vi "Find overlattice using co-incident search.vi"(6 "Minimal Angle from GB plane":dbl, 7 "Minimal thickness of the grain (A)":dbl=0.05, 8 "Co-incidence Tolerance":dbl=0.05, 9 "Number of integers to search":i32=50, 10 "Mutual Viewing Angle":dbl[](array[numeric])=[0.0, 1.0, 0.0], 11 "Grain Boundary Macro Definition":T1={"Grain 1 Orientation"=[1.0, 0.0, 0.0], "Grain 2 Orientation"=[0.707, 0.707, 0.0], "Twist Angle (Deg)"=0.0}) -> (1 "Perpendicular to GB Plane, Lattice c":dbl[](array[numeric]), 2 "GB Plane 2, Lattice b":dbl[](array[numeric]), 3 "GB Plane 1, Lattice a":dbl[](array[numeric]))   [LabVIEW 2010]
panel:
  out "Angle (Degrees)":dbl
  out "deleted portion":dbl[](array[numeric])
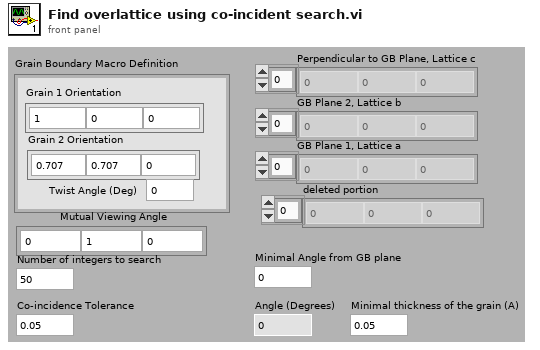
[diagram p1: front panel]
types:
  T1 = cluster{"Grain 1 Orientation":dbl[], "Grain 2 Orientation":dbl[], "Twist Angle (Deg)":dbl}
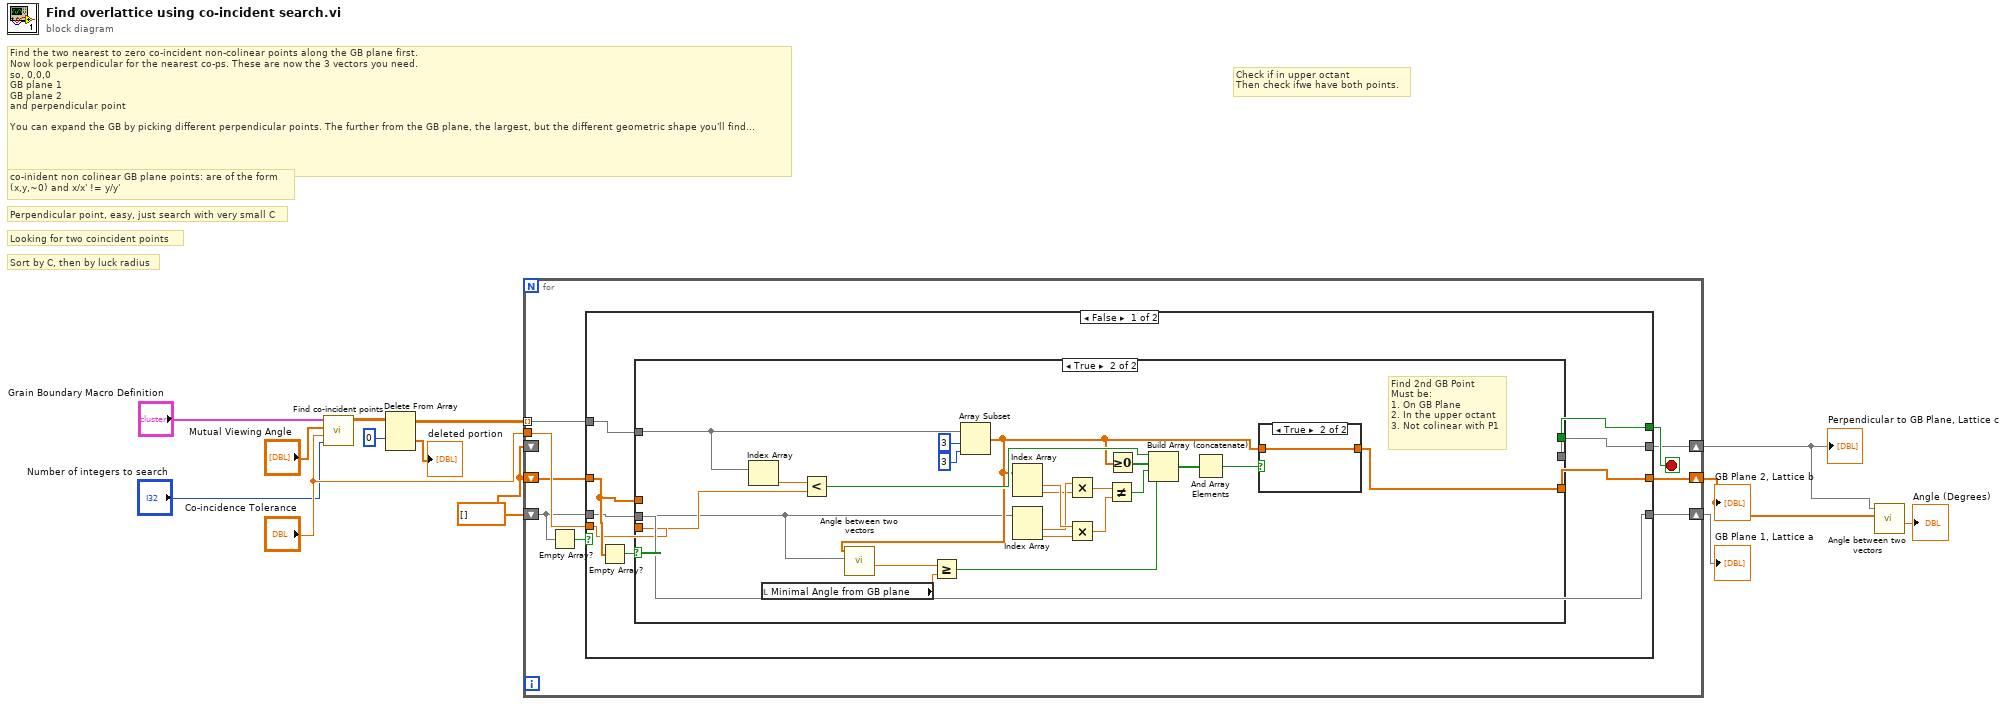
[diagram p0: block diagram]
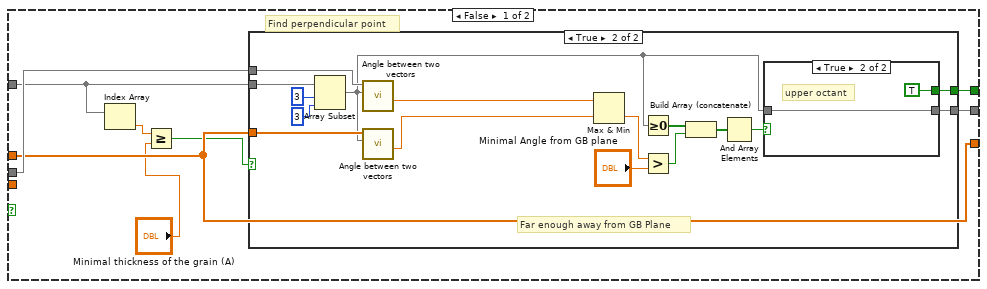
[diagram p2: hidden frame]
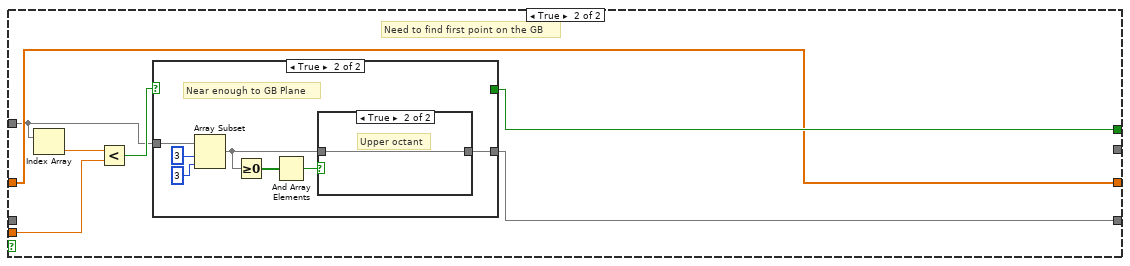
[diagram p6: hidden frame]
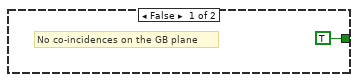
[diagram p7: hidden frame]
diagram:
  w9 = dbl[] []
  # "Check if in upper octant\nThen check ifwe have both points."
  # "Looking for two coincident points"
  # "Sort by C, then by luck radius"
  # "Perpendicular point, easy, just search with very small C"
  # "co-inident non colinear GB plane points: are of the form\n(x,y,~0) and x/x' != y/y'"
  # "Find the two nearest to zero co-incident non-colinear points along the GB plane first.\nNow look perpendicular for the nearest co-ps. These are now the 3 vectors you need. \nso, 0,0,0\nGB plane 1\nGB plane 2\nand perpendicular point\n\nYou can expand the GB by picking different perpendicular points. The further from the GB plane, the largest, but the different geometric shape you'll find..."
  n1 = call "Find co-incident points.vi"("Half of the number of integers to search"="Number of integers to search", "Co-incidence Tolerance"="Co-incidence Tolerance", "Mutual Viewing Angle"="Mutual Viewing Angle", "Grain Boundary Macro Definition"="Grain Boundary Macro Definition") -> ("Coincident points"=w12:dbl[][])  [unwired: 7 in]
  n2 = Delete From Array(array=w12, index (row)=0) -> (deleted portion=→"deleted portion":dbl[], array with subset deleted=w10:dbl[][])  [unwired: 2 in]
  n3 = for {
    tunnel: w10 -> [w14] mode=indexing
    shift-right: [w20] -> w5
    shift-left: w9 -> [w17]
    tunnel: "Co-incidence Tolerance" -> [w21]
    shift-right: [w16] -> w2
    shift-left: w9 -> [w18]
    shift-right: [w15] -> w3
    shift-left: w9 -> [_]
    stop <- w19 stop-if-true
    n4 = Empty Array?(array=w17) -> (empty?=w22:bool)
    n5 = case shown="False" w22 {
      tunnel: w14 -> [w24 w80]
      tunnel: w21 -> [w23 w85]
      tunnel: [w28 w83] -> w20
      tunnel: [w25 w82] -> w19
      tunnel: w18 -> [w29 w81]
      tunnel: w17 -> [w28 _]
      tunnel: [w27 w81] -> w16
      tunnel: [w26 _] -> w15
      frame False {
        n6 = Empty Array?(array=w29) -> (empty?=w30:bool)
        n7 = case shown="True" w30 {
          tunnel: w29 -> [w35 _]
          tunnel: w24 -> [w34 w65]
          tunnel: w28 -> [w36 w57]
          tunnel: [w35 w72] -> w27
          tunnel: w23 -> [_ w63]
          tunnel: [w38 _] -> w26
          tunnel: [w37 _] -> w25
          frame False {
            # "Find perpendicular point"
            n8 = Index Array(array=w34) -> (element=w33:dbl)  [unwired: 1 in]
            n9 = Greater Or Equal?(x=w33, y="Minimal thickness of the grain (A)") -> (x >= y?=w32:bool)
            n10 = case shown="True" w32 {
              tunnel: w34 -> [_ w51]
              tunnel: [_ w49] -> w38
              tunnel: [_ w52] -> w37
              tunnel: w36 -> [_ w48]
              tunnel: w35 -> [_ w47]
              frame False {
                # "Not far enough away from the GB Plane"
              }
              frame True {
                # "Far enough away from GB Plane"
                n11 = Array Subset(array=w51, index=3, length=3) -> (w39:dbl[])
                n12 = call "Angle between two vectors.vi"("Vector 2"=w39, "Vector 1"=w48) -> ("Angle (Degrees)"=w45:dbl)  [unwired: 7 in, 2 out]
                n13 = call "Angle between two vectors.vi"("Vector 2"=w39, "Vector 1"=w47) -> ("Angle (Degrees)"=w46:dbl)  [unwired: 7 in, 2 out]
                n14 = Max & Min(x=w45, y=w46) -> (min(x,y)=w44:dbl)  [unwired: 1 out]
                n15 = Greater Or Equal To 0?(x=w39) -> (x >= 0?=w41:bool[])
                n16 = Greater?(x=w44, y="Minimal Angle from GB plane") -> (0:w42:bool)
                n17 = Build Array (concatenate)(w41, w42) -> (w40:bool[])
                n18 = And Array Elements(Boolean array=w40) -> (logical AND=w50:bool)
                n19 = case shown="True" w50 {
                  tunnel: [_ TRUE] -> w52
                  tunnel: [_ w55] -> w49
                  tunnel: w39 -> [_ w55]
                  frame False {
                    # "elsewhere"
                  }
                  frame True {
                    # "upper octant"
                  }
                }
              }
            }
          }
          frame True {
            # "Find 2nd GB Point\nMust be:\n1. On GB Plane\n2. In the upper octant\n3. Not colinear with P1"
            n20 = Index Array(array=w65) -> (element=w64:dbl)  [unwired: 1 in]
            n21 = local read "Minimal Angle from GB plane"() -> (w60:dbl)
            n22 = Less?(x=w64, y=w63) -> (x < y?=w62:bool)
            n23 = Array Subset(array=w65, index=3, length=3) -> (w58:dbl[])
            n24 = call "Angle between two vectors.vi"("Vector 2"=w57, "Vector 1"=w58) -> ("Angle (Degrees)"=w61:dbl)  [unwired: 7 in, 2 out]
            n25 = Greater Or Equal?(x=w61, y=w60) -> (x >= y?=w59:bool)
            n26 = Index Array(array=w58) -> (element #1=w78:dbl, element #2=w75:dbl)  [unwired: 2 in]
            n27 = Index Array(array=w57) -> (element #1=w76:dbl, element #2=w77:dbl)  [unwired: 2 in]
            n28 = Multiply(x=w76, y=w75) -> (x*y=w74:dbl)
            n29 = Multiply(x=w78, y=w77) -> (x*y=w73:dbl)
            n30 = Not Equal?(x=w74, y=w73) -> (x != y?=w68:bool)
            n31 = Greater Or Equal To 0?(x=w58) -> (x >= 0?=w69:bool[])
            n32 = Build Array (concatenate)(w62, w69, w68, w59) -> (w67:bool[])
            n33 = And Array Elements(Boolean array=w67) -> (logical AND=w66:bool)
            n34 = case shown="True" w66 {
              tunnel: [_ w79] -> w72
              tunnel: w58 -> [_ w79]
              frame False {
                # "colinear"
              }
              frame True {
              }
            }
          }
        }
      }
      frame True {
        # "Need to find first point on the GB"
        n35 = Index Array(array=w80) -> (element=w86:dbl)  [unwired: 1 in]
        n36 = Less?(x=w86, y=w85) -> (x < y?=w84:bool)
        n37 = case shown="True" w84 {
          tunnel: w80 -> [_ w92]
          tunnel: [_ w88] -> w83
          tunnel: [TRUE _] -> w82
          frame False {
            # "No co-incidences on the GB plane"
          }
          frame True {
            # "Near enough to GB Plane"
            n38 = Array Subset(array=w92, index=3, length=3) -> (w89:dbl[])
            n39 = Greater Or Equal To 0?(x=w89) -> (x >= 0?=w91:bool[])
            n40 = And Array Elements(Boolean array=w91) -> (logical AND=w90:bool)
            n41 = case shown="True" w90 {
              tunnel: [_ w95] -> w88
              tunnel: w89 -> [_ w95]
              frame False {
                # "Elsewhere"
              }
              frame True {
                # "Upper octant"
              }
            }
          }
        }
      }
    }
  }
  "Perpendicular to GB Plane, Lattice c" <- w3
  "GB Plane 2, Lattice b" <- w2
  "GB Plane 1, Lattice a" <- w5
  n42 = call "Angle between two vectors.vi"("Vector 2"=w2, "Vector 1"=w3) -> ("Angle (Degrees)"=→"Angle (Degrees)":dbl)  [unwired: 7 in, 2 out]
